vi "main.vi"() -> ()   [LabVIEW 2017]
uses:
  VI Network cluster.ctl
panel:
  out "VI Total Network":T1[](array[typedef])
  out "VI Network":T1
  in  "Path":path
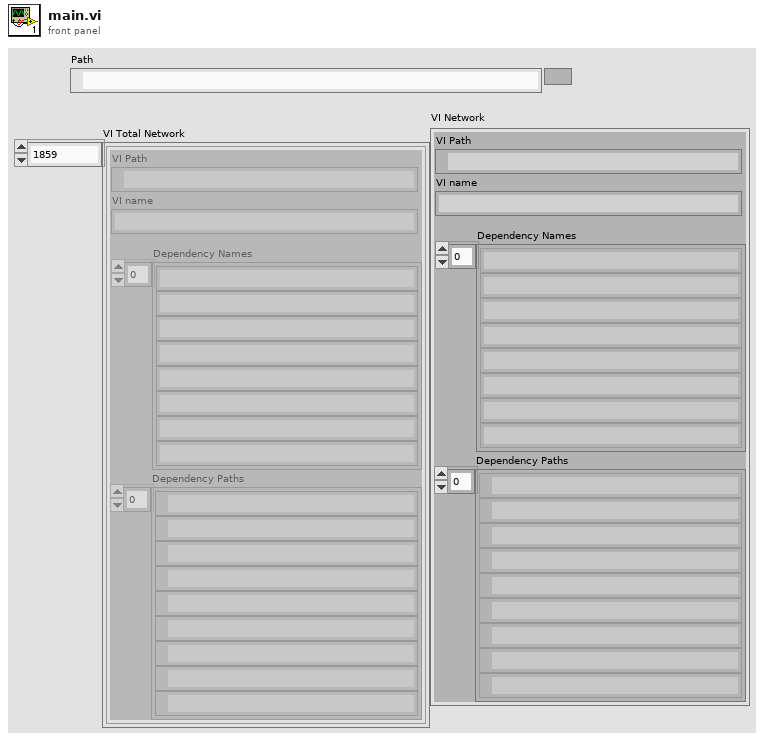
[diagram p1: front panel]
types:
  T1 = typedef "VI Network cluster.ctl" = cluster{"Dependency Names":string[], "Dependency Paths":path[], "VI Path":path, "VI name":string}
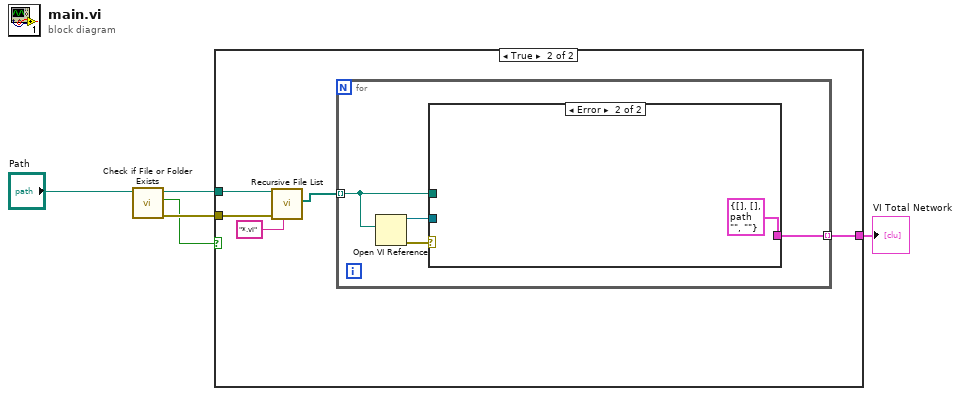
[diagram p0: block diagram]
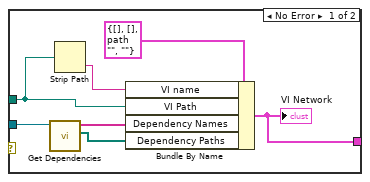
[diagram p3: hidden frame]
diagram:
  n1 = call <vilib>:"Check if File or Folder Exists.vi"("path"="Path") -> ("error out"=w5:errorcluster, "file or folder exists?"=w3:bool, "dup path"=w4:path)  [unwired: 8 in]
  n2 = case shown="True" w3 {
    tunnel: w5 -> [_ w10]
    tunnel: w4 -> [_ w9]
    tunnel: [_ w6] -> w1
    frame False {
    }
    frame True {
      n3 = call <vilib>:"Recursive File List.vi"("pattern"="*.vi", "error in (no error)"=w10, "Folder Path"=w9) -> ("All Files in Dir"=w8:path[])  [unwired: 4 in, 4 out]
      n4 = for {
        tunnel: w8 -> [w12] mode=indexing
        tunnel: [w11] -> w6 mode=indexing
        n5 = Open VI Reference(vi path=w12) -> (vi reference=w14:refnum<vi>, error out=w13:errorcluster)  [unwired: 5 in]
        n6 = case shown="Error" w13 {
          tunnel: w14 -> [w21 _]
          tunnel: w12 -> [w17 _]
          tunnel: [w15 T1 {"Dependency Names"=[], "Dependency Paths"=[], "VI Path"=path "", "VI name"=""} ("VI Network 2")] -> w11
          frame No Error {
            n7 = call "Get Dependencies.vi"("VI Refnum"=w21) -> ("Dependency Paths"=w19:path[], "Dependency Names"=w18:string[])  [unwired: 8 in, 1 out]
            n8 = Strip Path(path=w17) -> (name=w16:string)  [unwired: 1 out]
            n9 = Bundle By Name(cluster=T1 {"Dependency Names"=[], "Dependency Paths"=[], "VI Path"=path "", "VI name"=""} ("VI Network 2"), "VI name"=w16, "VI Path"=w17, "Dependency Names"=w18, "Dependency Paths"=w19) -> (w15:T1)
            "VI Network" <- w15
          }
          frame Error {
          }
        }
      }
    }
  }
  "VI Total Network" <- w1
